vi "测验程序4.vi"() -> ()   [LabVIEW 2017]
uses:
  <vilib>/userdefined/High Color/IMAQdx.ctl
  <vilib>/Platform/TimedLoop/XDataNode/timing_clust.ctl
  <vilib>/Platform/TimedLoop/XDataNode/nitl_modes.ctl
  <vilib>/Platform/TimedLoop/XDataNode/wakeup.ctl
  <vilib>/myRIO/Common/Instrument Driver Framework/myRIO v1.0/UART/vis/myRIO v1.0 Close UART.vi
  <vilib>/FPGAPlugInAG/myRIO-1900/niLvFpga_Open_myRIO-1900.vi
  <vilib>/rvi/interface/common/dynamic/niFpgaDynamicAddResources.vi
  <vilib>/myRIO/Common/Instrument Driver Framework/Utilities/vis/FPGA Ref Manager.vi
  <vilib>/Utility/error.llb/Error Cluster From Error Code.vi
  <vilib>/myRIO/Common/Instrument Driver Framework/Utilities/vis/Ref Counter.vi
  <vilib>/rvi/errors/niLvFpgaAdjustHostInterfaceError.vi
  <vilib>/FPGAPlugInAG/Dynamic/niLvFpga_Close_Dynamic.vi
  <vilib>/myRIO/Common/Instrument Driver Framework/myRIO v1.0/myRIO v1.0 Reset FPGA.vi
  <vilib>/myRIO/Common/Instrument Driver Framework/myRIO v1.0/IRQ/vis/myRIO v1.0 IRQ Info FGV.vi
  <vilib>/myRIO/Common/Instrument Driver Framework/myRIO v1.0/IRQ/vis/myRIO v1.0 Timer IRQ Info FGV.vi
  <vilib>/myRIO/Common/Instrument Driver Framework/myRIO v1.0/IRQ/vis/myRIO v1.0 ISR Agent.vi
  <vilib>/Platform/TimedLoop/XDataNode/XDataNode.xnode
  <vilib>/rvi/interface/nirviOpenFPGA/nirviOpenFPGA.xnode
  <vilib>/rvi/interface/nirviReadWriteControl/nirviReadWriteControl.xnode
  <vilib>/rvi/interface/nirviCloseFPGA/nirviCloseFPGA.xnode
  <vilib>/Platform/TimedLoop/XDataNode/XDNodeRunTimeDep.lvlib
  <vilib>/myRIO/Instrument Drivers/Utilities/Utilities.lvlib
  NiFpgaLv.dll
  <vilib>/rvi/interface/Simulation/niFpgaSimulationCallBeginRW.vi
  <vilib>/vision/driver/NI_Vision_Acquisition_Software.lvlib
  <vilib>/vision/NI_Vision_Development_Module.lvlib
panel:
  in  "Reset":bool
  in  "停止":bool
  out "数量":i32[](array[numeric])
  out "大小":dbl[](array[numeric])
  in  "保留图像？":bool
  in  "停止 2":bool
  out "货物类型":dbl
  in  "初始步态":u16
  in  "开始":bool
  in  "思币得":i32=60
  out "QTI":bool
  out "当前步态":u16
  out "超声波":u32[](array[numeric])
  # "4小蓝"
  # "3小红"
  # "2大蓝"
  # "100000"
  # "1大红"
  # "70000"
  # "0异常"
  # "14600夹取高度"
  # "25000"
  # "700夹住"
  # "-1010"
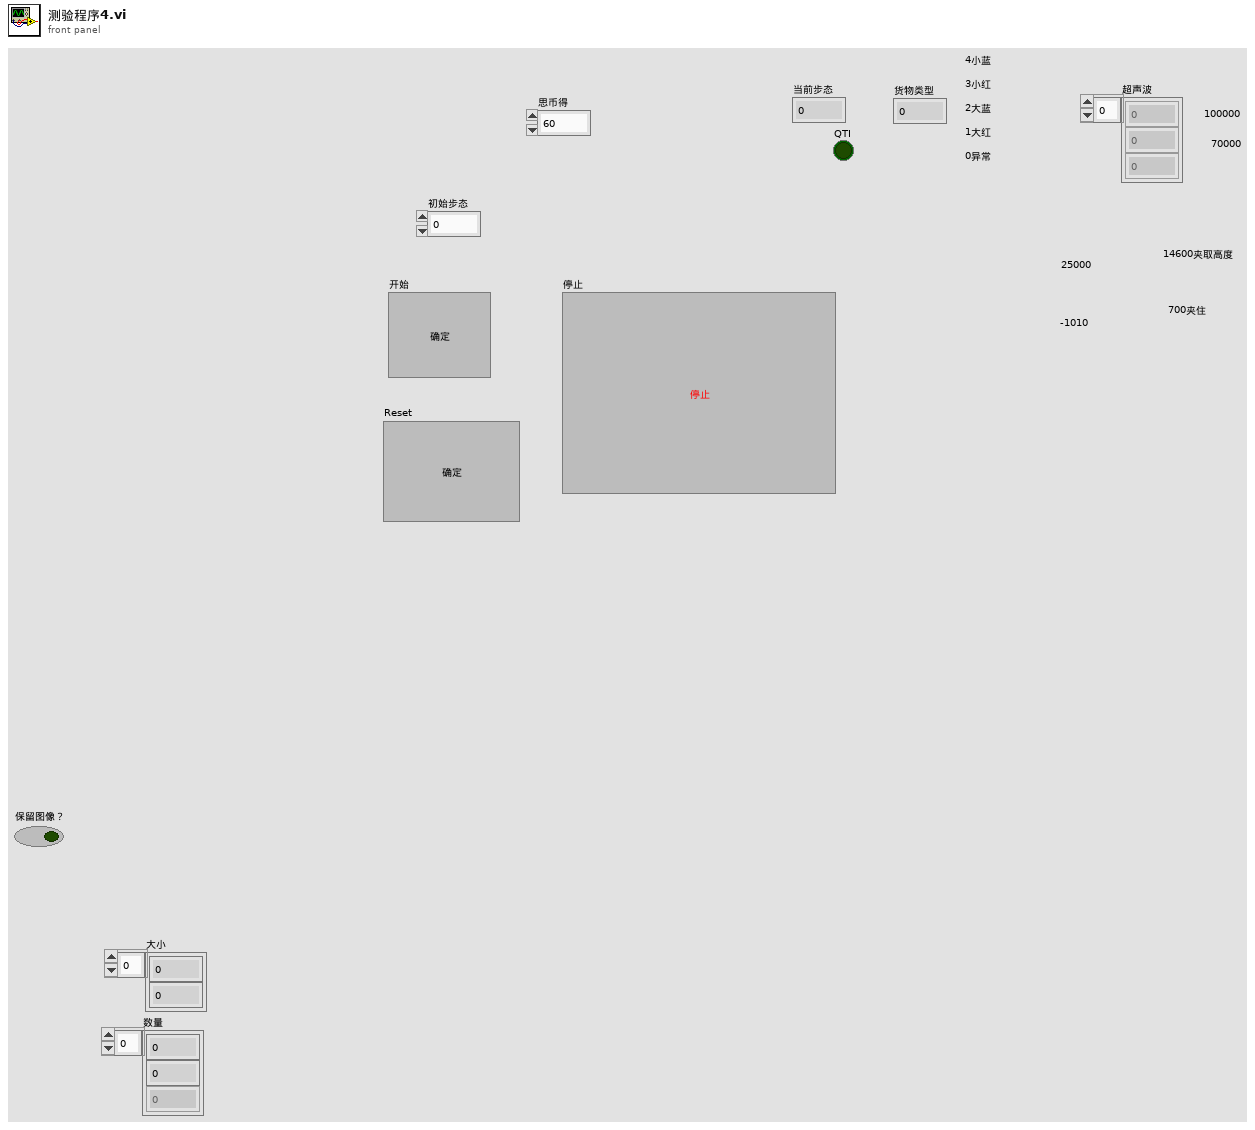
[diagram p1: front panel]
types:
  T1 = typedef "IMAQdx.ctl" = refnum<k21>
  T2 = typedef "IMAQ Image.ctl" = refnum<image>
  T3 = typedef "XDNodeRunTimeDep.lvlib/timing_clust.ctl" = cluster{"Expected End [f-1]":u64, "Actual End [f-1]":u64, "Finished Late? [f-1]":bool, "Expected End [i-1]":u64, "Actual End [i-1]":u64, "Finished Late? [i-1]":bool, "Expected Start [i]":u64, "Actual Start [i]":u64, "Expected Start [f]":u64, "Actual Start [f]":u64, "Source Name":string, "Structure Name":string, "Period":i64, "Deadline":i64, "Offset":i64, "Start":i64, "Priority":i32, "Timeout":i32, "Mode":T4, "Wakeup Reason":T5, "Error":errorcluster, "Source Type":string, "Secondary Source Type":string, "Global End Time":u64, "Global Start Time":u64, "Frame Duration":u64, "Iteration Duration":u64, "Assigned CPU":i32, "I/O Scan Engine Mode":u32}
  T4 = typedef "XDNodeRunTimeDep.lvlib/nitl_modes.ctl" = enum32{"No Change", "Process missed periods, maintain original phase", "Discard missed periods, maintain original phase", "Process missed periods, ignore original phase", "Discard missed periods, ignore original phase"}
  T5 = typedef "XDNodeRunTimeDep.lvlib/wakeup.ctl" = enum32{"Normal", "Aborted", "Asynchronous wakeup", "Timing source error", "Timed loop error", "Timeout"}
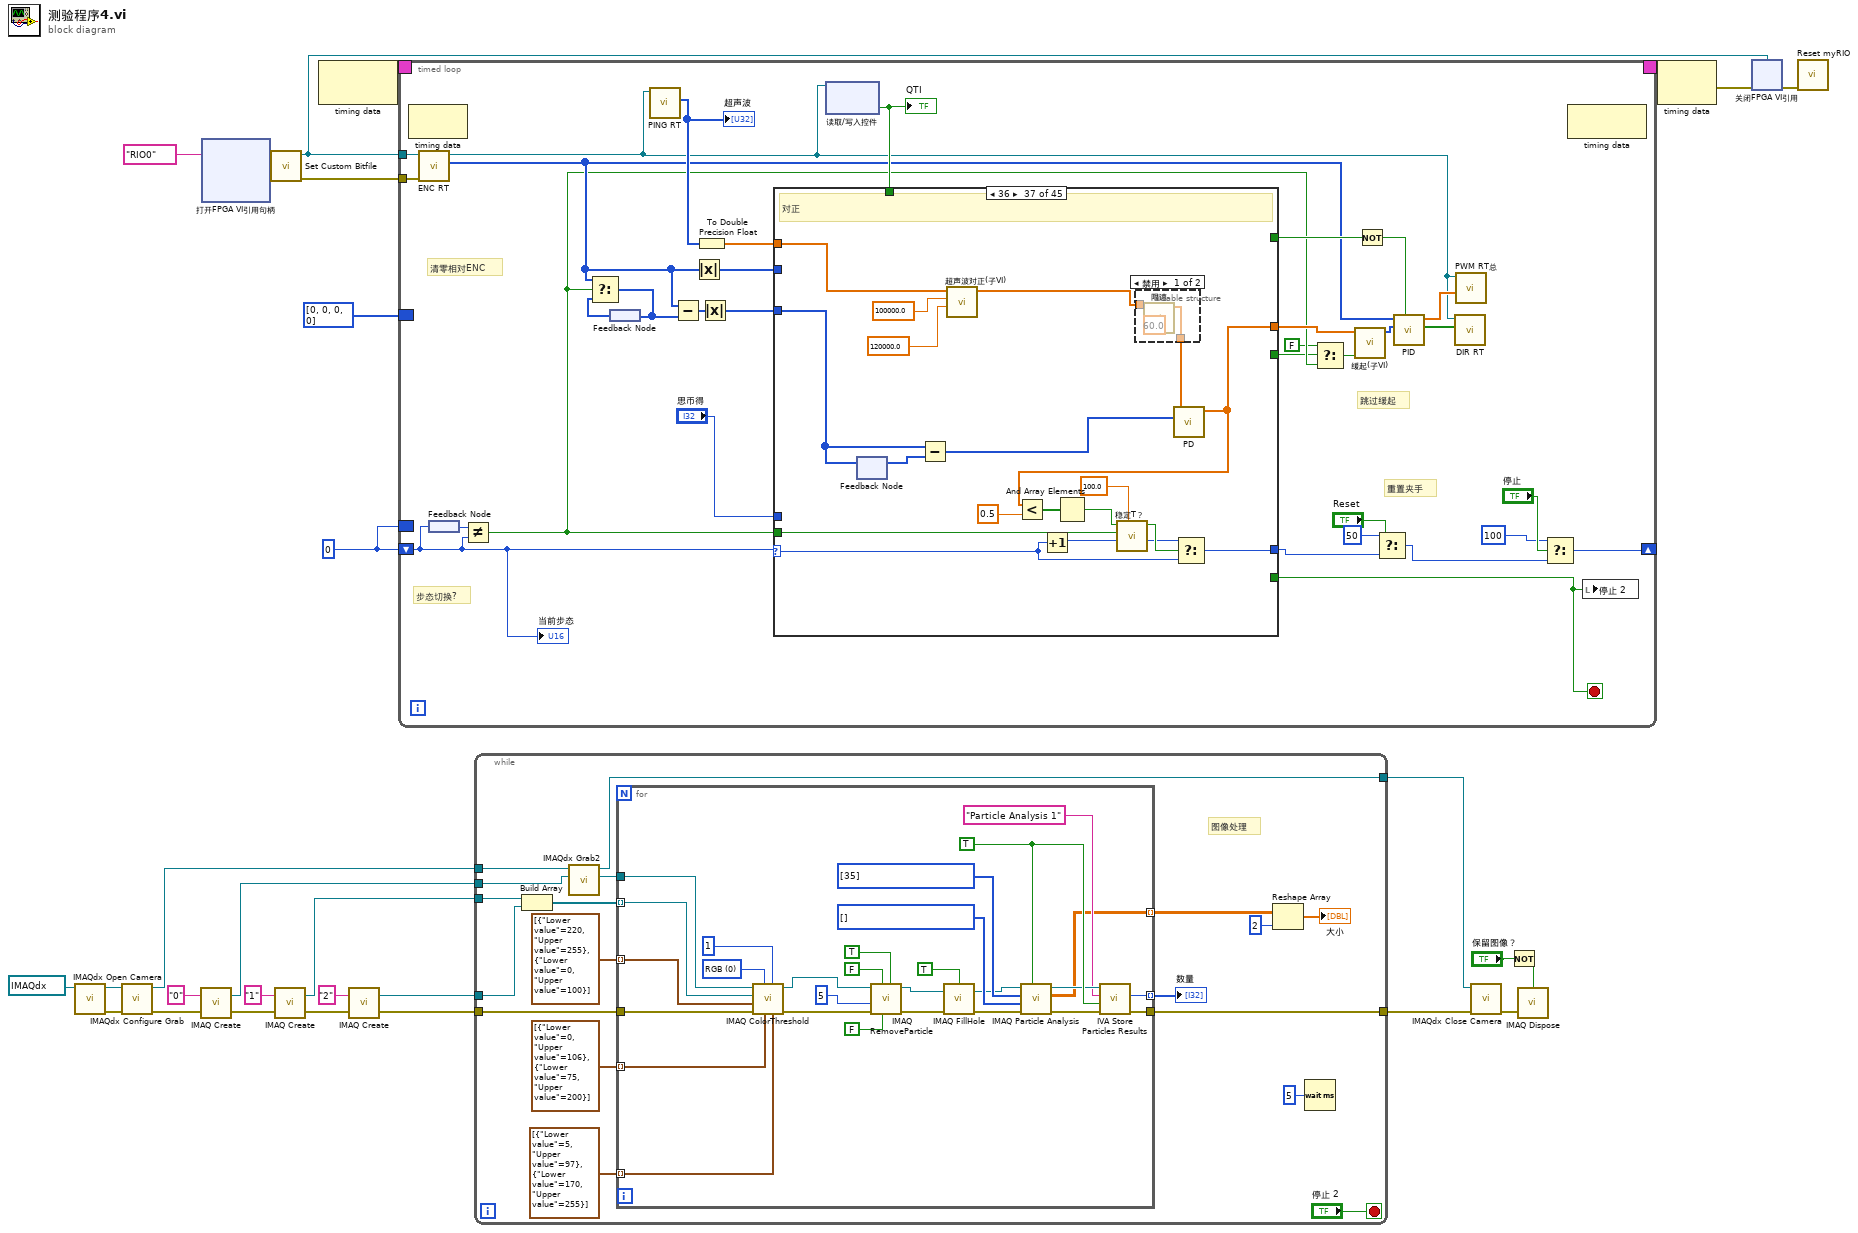
[diagram p0: block diagram]
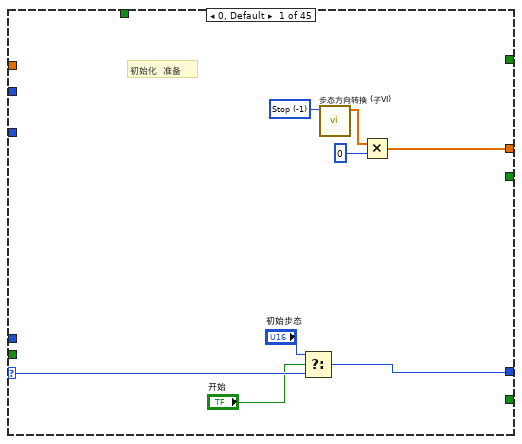
[diagram p2: hidden frame]
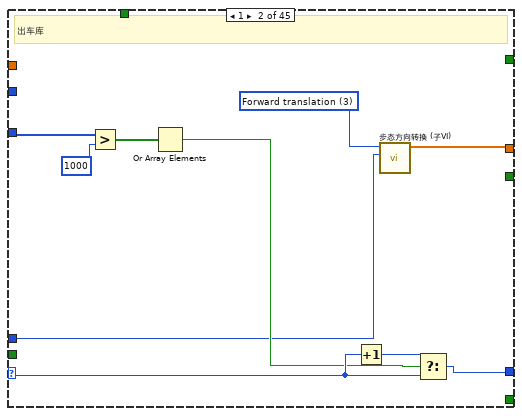
[diagram p3: hidden frame]
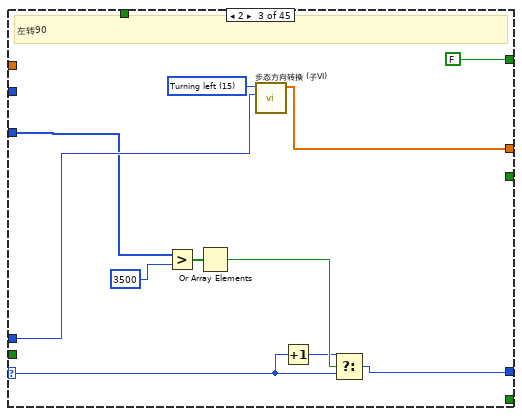
[diagram p4: hidden frame]
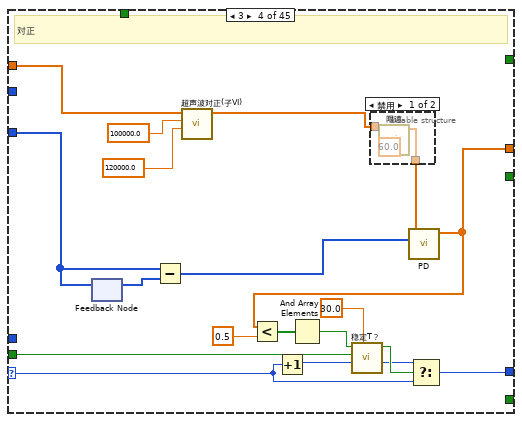
[diagram p5: hidden frame]
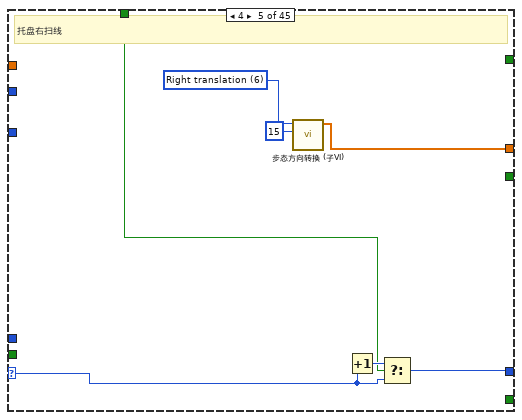
[diagram p7: hidden frame]
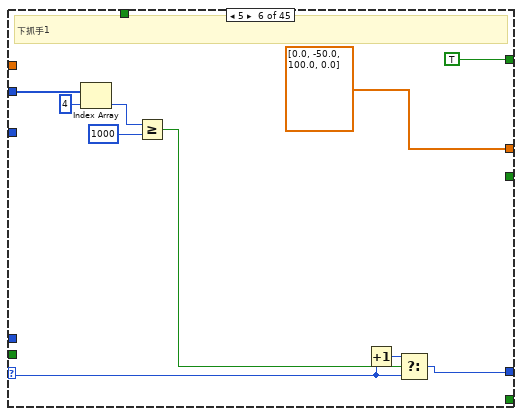
[diagram p8: hidden frame]
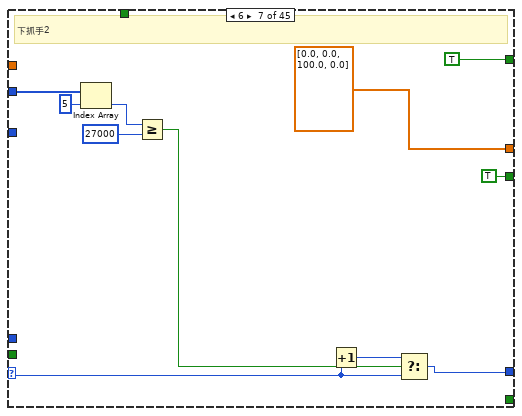
[diagram p9: hidden frame]
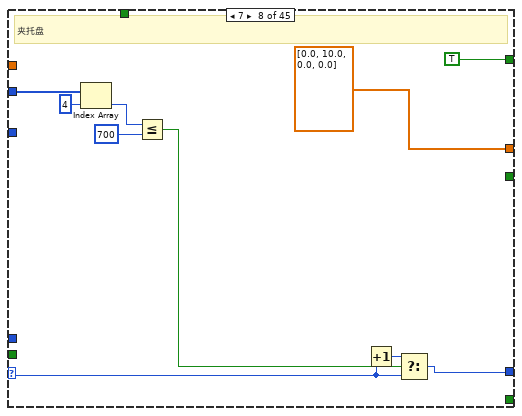
[diagram p10: hidden frame]
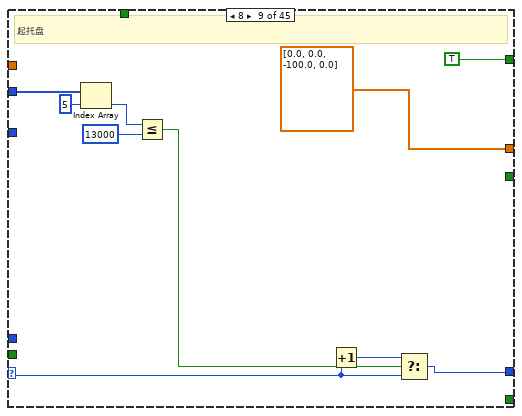
[diagram p11: hidden frame]
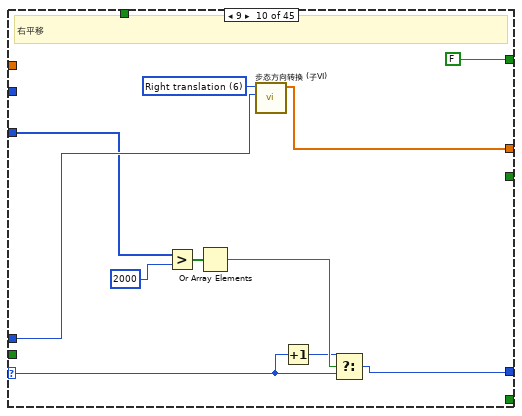
[diagram p12: hidden frame]
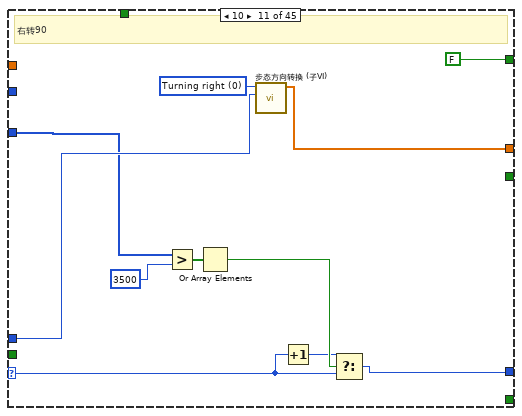
[diagram p13: hidden frame]
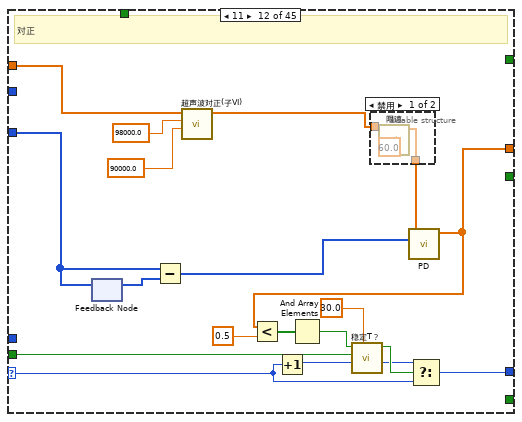
[diagram p14: hidden frame]
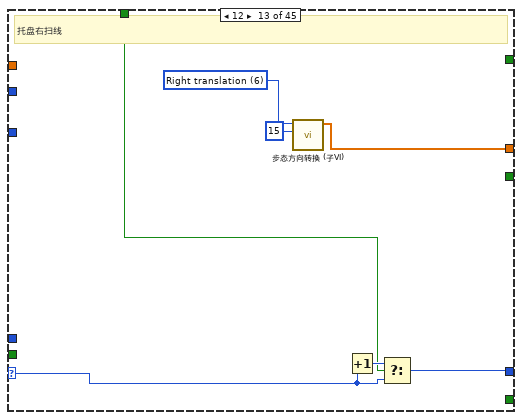
[diagram p16: hidden frame]
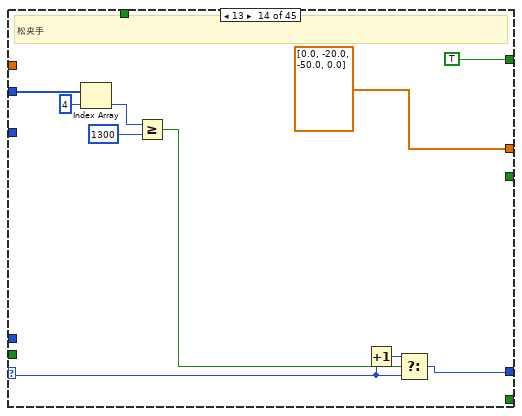
[diagram p17: hidden frame]
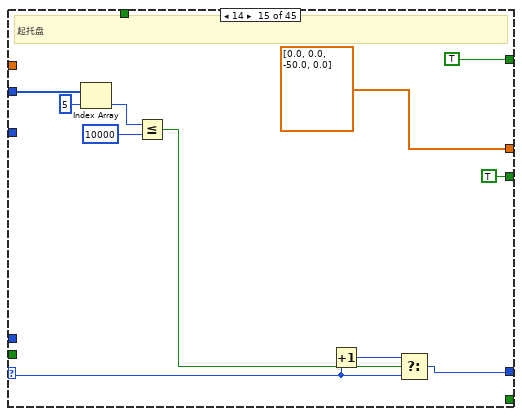
[diagram p18: hidden frame]
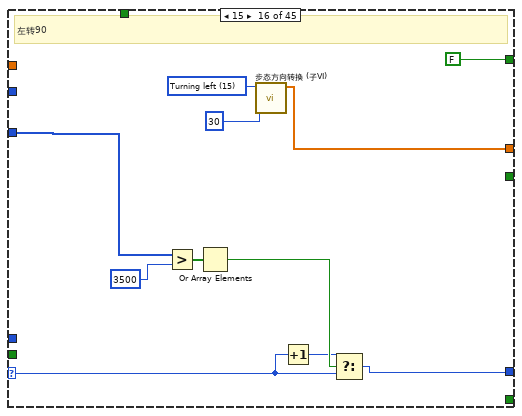
[diagram p19: hidden frame]
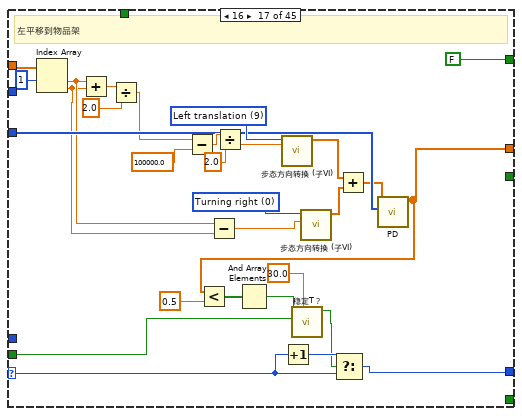
[diagram p20: hidden frame]
diagram:
  w28 = u16 0 ("初始步态")
  n1 = call <vilib>:"IMAQdx Open Camera.vi"("Session In"=T1 "cam0") -> ("error out"=w15:errorcluster, "Session Out"=w14:T1)  [unwired: 9 in]
  n2 = call <vilib>:"IMAQdx Configure Grab.vi"("error in"=w15, "Session In"=w14) -> ("error out"=w12:errorcluster, "Session Out"=w19:T1)  [unwired: 8 in]
  n3 = call "IMAQ Create"("Image Name"="0", "error in (no error)"=w12) -> ("New Image"=w17:T2, "error out"=w10:errorcluster)  [unwired: 3 in]
  n4 = xnode "打开FPGA VI引用句柄"("资源名称"=tag "RIO0") -> ("FPGA VI引用输出"=w24:refnum<k20>, "错误输出"=w23:errorcluster)  [unwired: 1 in]
  n5 = call <vilib>:"Set Custom Bitfile.vi"("error in (no error)"=w23, "Custom FPGA Reference In"=w24) -> ("error out"=w22:errorcluster, "Custom FPGA Reference Out"=w20:refnum<k20>)  [unwired: 8 in]
  n6 = call "IMAQ Create"("Image Name"="1", "error in (no error)"=w10) -> ("New Image"=w7:T2, "error out"=w8:errorcluster)  [unwired: 3 in]
  n7 = node-c288() -> (w30:T3)  [unwired: 1 in]
  n8 = call "IMAQ Create"("Image Name"="2", "error in (no error)"=w8) -> ("New Image"=w6:T2, "error out"=w5:errorcluster)  [unwired: 3 in]
  n9 = timed-loop {
    timing: w30 -> [_]
    timing-out: [_] -> w29
    shift-right: [w42] -> _
    shift-left: w28 -> [w31]
    border: w28 -> [_]
    border: i32[] [0, 0, 0, 0] ("ENC") -> [_]
    tunnel: w22 -> [w60]
    tunnel: w20 -> [w57]
    stop <- w43 stop-if-true
    # "重置夹手"
    # "跳过缓起"
    # "步态切换?"
    # "清零相对ENC"
    n10 = node-c288() -> ()  [unwired: 1 in, 1 out]
    n11 = call "ENC RT.vi"("错误输入（无错误）"=w60, "Custom FPGA Reference Out"=w57) -> ("ENC"=w47:i32[], "FPGA VI引用输出"=w45:refnum<k20>)  [unwired: 7 in, 1 out]
    n12 = feedback-in #1(w31) -> ()
    n13 = feedback #1() -> (w61:u16)
    n14 = Not Equal?(x=w61, y=w31) -> (x != y?=w35:bool)
    n15 = feedback #2() -> (w59:i32[])
    n16 = Select(t=w47, s=w35, f=w59) -> (s? t:f=w44:i32[])
    n17 = feedback-in #2(w44) -> ()
    n18 = call "PING RT.vi"("引用句柄输入"=w45) -> ("PING"=w51:u32[])  [unwired: 8 in, 2 out]
    "超声波" <- w51
    n19 = Subtract(x=w47, y=w44) -> (x-y=w52:i32[])
    n20 = Absolute Value(x=w47) -> (abs(x)=w46:i32[])
    n21 = To Double Precision Float(number=w51) -> (double precision float=w50:dbl[])
    n22 = Absolute Value(x=w52) -> (abs(x)=w48:i32[])
    n23 = xnode "读取/写入控件"("FPGA VI引用输入"=w45) -> ("QTI"=w49:bool)  [unwired: 1 in, 2 out]
    "QTI" <- w49
    n24 = case shown="36" w31 {
      selector: w31 -> [w68 w74 w85 w108 w118 w128 w140 w150 w160 w166 w177 w200 w210 w221 w232 w239 w272 w278 w286 w310 w316 w327 w337 w347 w353 w387 w393 w401 w423 w429 w440 w451 w462 w472 w479 w488 w511 w526 w536 w545 w557 w568 w579 w587 w599]
      tunnel: [w69 w81 w86 w102 w119 dbl[] [0.0, -50.0, 100.0, 0.0] ("输出") dbl[] [0.0, 0.0, 100.0, 0.0] ("输出") dbl[] [0.0, 10.0, 0.0, 0.0] ("输出") dbl[] [0.0, 0.0, -100.0, 0.0] ("输出") w167 w178 w194 w211 dbl[] [0.0, -20.0, -50.0, 0.0] ("输出") dbl[] [0.0, 0.0, -50.0, 0.0] ("输出") w240 w260 w279 w287 w297 w317 dbl[] [0.0, 0.0, 50.0, 0.0] ("输出") dbl[] [0.0, 10.0, 0.0, 0.0] ("输出") dbl[] [0.0, 0.0, -50.0, 0.0] ("输出") w354 w375 w394 w402 w411 w430 dbl[] [0.0, -10.0, 0.0, 0.0] ("输出") dbl[] [0.0, 0.0, 100.0, 0.0] ("输出") dbl[] [0.0, 10.0, 0.0, 0.0] ("输出") dbl[] [0.0, 0.0, -100.0, 0.0] ("输出") w480 w495 w505 dbl[] [0.0, 0.0, 100.0, 0.0] ("输出") dbl[] [0.0, -10.0, 0.0, 0.0] ("输出") dbl[] [0.0, 50.0, -100.0, 0.0] ("输出") dbl[] [0.0, 0.0, -100.0, 0.0] ("输出") w566 dbl[] [0.0, 10.0, 0.0, 0.0] ("输出") dbl[] [0.0, 0.0, 0.0, 0.0] ("输出") dbl[] [0.0, 0.0, 0.0, 0.0] ("输出")] -> w56
      tunnel: "思币得" -> [_ w72 w87 _ _ _ _ _ _ w168 w179 _ _ _ _ _ _ _ _ _ _ _ _ _ w355 _ _ _ _ _ _ _ _ _ _ _ _ _ _ _ _ w560 _ _ _]
      tunnel: [w66 w77 w92 w107 w116 w130 w141 w151 w161 w173 w184 w199 w208 w222 w233 w245 w274 w276 w292 w312 w314 w328 w338 w348 w360 w389 w391 w407 w425 w427 w441 w452 w463 w473 w485 w491 w510 w527 w537 w547 w558 w569 w581 w589 w599] -> w39
      tunnel: [_ _ FALSE ("继电器") _ _ TRUE ("继电器") TRUE ("继电器") TRUE ("继电器") TRUE ("继电器") FALSE ("继电器") FALSE ("继电器") _ _ TRUE ("继电器") TRUE ("继电器") FALSE ("继电器") FALSE ("继电器") _ FALSE ("继电器") FALSE ("继电器") _ TRUE ("继电器") TRUE ("继电器") TRUE ("继电器") FALSE ("继电器") FALSE ("继电器") _ FALSE ("继电器") FALSE ("继电器") _ TRUE ("继电器") TRUE ("继电器") TRUE ("继电器") TRUE ("继电器") FALSE ("继电器") _ _ TRUE ("继电器") TRUE ("继电器") TRUE ("继电器") TRUE ("继电器") _ TRUE ("继电器") _ _] -> w54
      tunnel: w48 -> [_ w79 w83 w105 _ _ _ _ _ w164 w175 w197 _ _ _ w237 w266 _ w284 w303 _ _ _ _ w351 w381 _ w399 w417 _ _ _ _ _ w477 w493 w508 _ _ _ _ w562 _ _ _]
      tunnel: w50 -> [_ _ _ w110 _ _ _ _ _ _ _ w202 _ _ _ _ w270 _ _ w308 _ _ _ _ _ w385 _ _ w421 _ _ _ _ _ _ _ w513 _ _ _ _ _ _ _ _]
      tunnel: w35 -> [_ _ _ w97 _ _ _ _ _ _ _ w189 _ _ _ _ w259 _ _ w296 _ _ _ _ _ w374 _ _ w410 _ _ _ _ _ _ _ w500 _ _ _ _ _ _ _ _]
      tunnel: w49 -> [_ _ _ _ w115 _ _ _ _ _ _ _ w207 _ _ _ _ w275 _ _ w313 _ _ _ _ _ w390 _ _ w426 _ _ _ _ _ _ _ _ _ _ _ _ _ _ _]
      tunnel: w46 -> [_ _ _ _ _ w122 w134 w144 w154 _ _ _ _ w215 w226 _ _ _ _ _ _ w321 w331 w341 _ _ _ _ _ _ w434 w445 w456 w466 _ _ _ w520 w530 w539 w551 _ w573 _ _]
      tunnel: [_ _ _ _ _ _ _ _ _ _ _ _ _ _ _ _ _ _ _ _ _ _ _ _ _ _ _ _ _ _ _ _ _ _ _ _ _ _ _ _ _ _ _ _ TRUE ("停止 2")] -> w43
      tunnel: [_ _ _ _ _ _ TRUE ("t") _ _ _ _ _ _ _ TRUE ("t") _ _ _ _ _ _ _ _ _ _ _ _ _ _ _ _ TRUE ("t") TRUE ("t") _ _ _ _ TRUE ("t") _ _ TRUE ("t") _ _ _ _] -> w32
      frame 0, Default {
        w71 = i8 -1 items=["Stop"=-1, "Right translation"=6, "Back translation"=12, "Turning right"=0, "Turning left"=15, "Forward translation"=3, "Left translation"=9, "Gyro rotating"=16] ("Gait")
        # "初始化  准备"
        n25 = Select(t="初始步态", s="开始", f=w68) -> (s? t:f=w66:u16)
        n26 = call "步态方向转换 (子VI).vi"("Gait"=w71) -> ("输出"=w70:dbl[])  [unwired: 10 in]
        n27 = Multiply(x=w70, y=0 ("长度")) -> (x*y=w69:dbl[])
      }
      frame 1 {
        w80 = i8 3 items=["Stop"=-1, "Right translation"=6, "Back translation"=12, "Turning right"=0, "Turning left"=15, "Forward translation"=3, "Left translation"=9, "Gyro rotating"=16] ("Gait")
        # "出车库"
        n28 = Greater?(x=w79, y=1000) -> (0:w76:bool[])
        n29 = Or Array Elements(Boolean array=w76) -> (logical OR=w73:bool)
        n30 = Increment(x=w74) -> (x+1=w75:u16)
        n31 = call "步态方向转换 (子VI).vi"("速度"=w72, "Gait"=w80) -> ("输出"=w81:dbl[])  [unwired: 9 in]
        n32 = Select(t=w75, s=w73, f=w74) -> (s? t:f=w77:u16)
      }
      frame 2 {
        w88 = i8 15 items=["Stop"=-1, "Right translation"=6, "Back translation"=12, "Turning right"=0, "Turning left"=15, "Forward translation"=3, "Left translation"=9, "Gyro rotating"=16] ("Gait")
        # "左转90"
        n33 = Greater?(x=w83, y=3500 ("次数")) -> (0:w90:bool[])
        n34 = Or Array Elements(Boolean array=w90) -> (logical OR=w89:bool)
        n35 = call "步态方向转换 (子VI).vi"("速度"=w87, "Gait"=w88) -> ("输出"=w86:dbl[])  [unwired: 9 in]
        n36 = Increment(x=w85) -> (x+1=w84:u16)
        n37 = Select(t=w84, s=w89, f=w85) -> (s? t:f=w92:u16)
      }
      frame 3 {
        # "对正"
        n38 = feedback-in #3(w105) -> ()
        n39 = feedback #3() -> (w104:i32[])  [unwired: 1 in]
        n40 = Subtract(x=w105, y=w104) -> (x-y=w103:i32[])
        n41 = call "超声波对正(子VI).vi"("LFT"=120000.0, "FWD"=100000.0, "数组输入"=w110) -> ("数组输出"=w109:dbl[])  [unwired: 8 in]
        n42 = Increment(x=w108) -> (x+1=w93:u16)
        n43 = disable-structure shown="禁用" {
          disable-tunnel: w109 -> [w113 w114]
          disable-tunnel: [w111 w114] -> w106
          frame Disabled {
            n44 = call "限速.vi"("最大值"=60.0, "输入"=w113) -> ("数组"=w111:dbl[])  [unwired: 9 in]
          }
          frame Enabled {
          }
        }
        n45 = call "PD.vi"("ENC"=w103, "SET"=w106) -> ("output"=w102:dbl[])  [unwired: 9 in]
        n46 = Less?(x=w102, y=0.5) -> (x < y?=w100:bool[])
        n47 = And Array Elements(Boolean array=w100) -> (logical AND=w99:bool)
        n48 = call "稳定T？.vi"("次数(100)"=30.0, "Reset"=w97, "输入"=w99) -> ("TT？"=w98:bool)  [unwired: 8 in]
        n49 = Select(t=w93, s=w98, f=w108) -> (s? t:f=w107:u16)
      }
      frame 4 {
        w121 = i8 6 items=["Stop"=-1, "Right translation"=6, "Back translation"=12, "Turning right"=0, "Turning left"=15, "Forward translation"=3, "Left translation"=9, "Gyro rotating"=16] ("Gait")
        # "托盘右扫线"
        n50 = call "步态方向转换 (子VI).vi"("速度"=15, "Gait"=w121) -> ("输出"=w119:dbl[])  [unwired: 9 in]
        n51 = Increment(x=w118) -> (x+1=w117:u16)
        n52 = Select(t=w117, s=w115, f=w118) -> (s? t:f=w116:u16)
      }
      frame 5 {
        # "下抓手1"
        n53 = Index Array(array=w122, index=4 ("索引")) -> (element=w125:i32)
        n54 = Greater Or Equal?(x=w125, y=1000) -> (x >= y?=w123:bool)
        n55 = Increment(x=w128) -> (x+1=w129:u16)
        n56 = Select(t=w129, s=w123, f=w128) -> (s? t:f=w130:u16)
      }
      frame 6 {
        # "下抓手2"
        n57 = Index Array(array=w134, index=5 ("索引")) -> (element=w137:i32)
        n58 = Greater Or Equal?(x=w137, y=27000) -> (x >= y?=w135:bool)
        n59 = Increment(x=w140) -> (x+1=w133:u16)
        n60 = Select(t=w133, s=w135, f=w140) -> (s? t:f=w141:u16)
      }
      frame 7 {
        # "夹托盘"
        n61 = Index Array(array=w144, index=4 ("索引")) -> (element=w147:i32)
        n62 = Less Or Equal?(x=w147, y=700) -> (x <= y?=w145:bool)
        n63 = Increment(x=w150) -> (x+1=w143:u16)
        n64 = Select(t=w143, s=w145, f=w150) -> (s? t:f=w151:u16)
      }
      frame 8 {
        # "起托盘"
        n65 = Index Array(array=w154, index=5 ("索引")) -> (element=w157:i32)
        n66 = Less Or Equal?(x=w157, y=13000) -> (x <= y?=w155:bool)
        n67 = Increment(x=w160) -> (x+1=w153:u16)
        n68 = Select(t=w153, s=w155, f=w160) -> (s? t:f=w161:u16)
      }
      frame 9 {
        w169 = i8 6 items=["Stop"=-1, "Right translation"=6, "Back translation"=12, "Turning right"=0, "Turning left"=15, "Forward translation"=3, "Left translation"=9, "Gyro rotating"=16] ("Gait")
        # "右平移"
        n69 = Greater?(x=w164, y=2000 ("次数")) -> (0:w171:bool[])
        n70 = Or Array Elements(Boolean array=w171) -> (logical OR=w170:bool)
        n71 = call "步态方向转换 (子VI).vi"("速度"=w168, "Gait"=w169) -> ("输出"=w167:dbl[])  [unwired: 9 in]
        n72 = Increment(x=w166) -> (x+1=w165:u16)
        n73 = Select(t=w165, s=w170, f=w166) -> (s? t:f=w173:u16)
      }
      frame 10 {
        w180 = i8 0 items=["Stop"=-1, "Right translation"=6, "Back translation"=12, "Turning right"=0, "Turning left"=15, "Forward translation"=3, "Left translation"=9, "Gyro rotating"=16] ("Gait")
        # "右转90"
        n74 = Greater?(x=w175, y=3500 ("次数")) -> (0:w182:bool[])
        n75 = Or Array Elements(Boolean array=w182) -> (logical OR=w181:bool)
        n76 = call "步态方向转换 (子VI).vi"("速度"=w179, "Gait"=w180) -> ("输出"=w178:dbl[])  [unwired: 9 in]
        n77 = Increment(x=w177) -> (x+1=w176:u16)
        n78 = Select(t=w176, s=w181, f=w177) -> (s? t:f=w184:u16)
      }
      frame 11 {
        # "对正"
        n79 = feedback-in #4(w197) -> ()
        n80 = feedback #4() -> (w196:i32[])  [unwired: 1 in]
        n81 = Subtract(x=w197, y=w196) -> (x-y=w195:i32[])
        n82 = call "超声波对正(子VI).vi"("LFT"=90000.0, "FWD"=98000.0, "数组输入"=w202) -> ("数组输出"=w201:dbl[])  [unwired: 8 in]
        n83 = Increment(x=w200) -> (x+1=w185:u16)
        n84 = disable-structure shown="禁用" {
          disable-tunnel: w201 -> [w205 w206]
          disable-tunnel: [w203 w206] -> w198
          frame Disabled {
            n85 = call "限速.vi"("最大值"=60.0, "输入"=w205) -> ("数组"=w203:dbl[])  [unwired: 9 in]
          }
          frame Enabled {
          }
        }
        n86 = call "PD.vi"("ENC"=w195, "SET"=w198) -> ("output"=w194:dbl[])  [unwired: 9 in]
        n87 = Less?(x=w194, y=0.5) -> (x < y?=w192:bool[])
        n88 = And Array Elements(Boolean array=w192) -> (logical AND=w191:bool)
        n89 = call "稳定T？.vi"("次数(100)"=30.0, "Reset"=w189, "输入"=w191) -> ("TT？"=w190:bool)  [unwired: 8 in]
        n90 = Select(t=w185, s=w190, f=w200) -> (s? t:f=w199:u16)
      }
      frame 12 {
        w213 = i8 6 items=["Stop"=-1, "Right translation"=6, "Back translation"=12, "Turning right"=0, "Turning left"=15, "Forward translation"=3, "Left translation"=9, "Gyro rotating"=16] ("Gait")
        # "托盘右扫线"
        n91 = call "步态方向转换 (子VI).vi"("速度"=15, "Gait"=w213) -> ("输出"=w211:dbl[])  [unwired: 9 in]
        n92 = Increment(x=w210) -> (x+1=w209:u16)
        n93 = Select(t=w209, s=w207, f=w210) -> (s? t:f=w208:u16)
      }
      frame 13 {
        # "松夹手"
        n94 = Index Array(array=w215, index=4 ("索引")) -> (element=w218:i32)
        n95 = Greater Or Equal?(x=w218, y=1300) -> (x >= y?=w216:bool)
        n96 = Increment(x=w221) -> (x+1=w214:u16)
        n97 = Select(t=w214, s=w216, f=w221) -> (s? t:f=w222:u16)
      }
      frame 14 {
        # "起托盘"
        n98 = Index Array(array=w226, index=5 ("索引")) -> (element=w229:i32)
        n99 = Less Or Equal?(x=w229, y=10000) -> (x <= y?=w227:bool)
        n100 = Increment(x=w232) -> (x+1=w225:u16)
        n101 = Select(t=w225, s=w227, f=w232) -> (s? t:f=w233:u16)
      }
      frame 15 {
        w241 = i8 15 items=["Stop"=-1, "Right translation"=6, "Back translation"=12, "Turning right"=0, "Turning left"=15, "Forward translation"=3, "Left translation"=9, "Gyro rotating"=16] ("Gait")
        # "左转90"
        n102 = Greater?(x=w237, y=3500 ("次数")) -> (0:w243:bool[])
        n103 = Or Array Elements(Boolean array=w243) -> (logical OR=w242:bool)
        n104 = call "步态方向转换 (子VI).vi"("速度"=30, "Gait"=w241) -> ("输出"=w240:dbl[])  [unwired: 9 in]
        n105 = Increment(x=w239) -> (x+1=w238:u16)
        n106 = Select(t=w238, s=w242, f=w239) -> (s? t:f=w245:u16)
      }
      frame 16 {
        w251 = i8 0 items=["Stop"=-1, "Right translation"=6, "Back translation"=12, "Turning right"=0, "Turning left"=15, "Forward translation"=3, "Left translation"=9, "Gyro rotating"=16] ("Gait")
        w269 = i8 9 items=["Stop"=-1, "Right translation"=6, "Back translation"=12, "Turning right"=0, "Turning left"=15, "Forward translation"=3, "Left translation"=9, "Gyro rotating"=16] ("Gait")
        # "左平移到物品架"
        n107 = Index Array(array=w270, index #1=1 ("索引")) -> (element #1=w250:dbl, element #2=w249:dbl)  [unwired: 1 in]
        n108 = Add(x=w250, y=w249) -> (x+y=w255:dbl)
        n109 = Divide(x=w255, y=2.0) -> (x/y=w253:dbl)
        n110 = Subtract(x=w253, y=100000.0) -> (x-y=w268:dbl)
        n111 = Subtract(x=w250, y=w249) -> (x-y=w252:dbl)
        n112 = Divide(x=w268, y=2.0 ("x")) -> (x/y=w258:dbl)
        n113 = call "步态方向转换 (子VI).vi"("速度"=w258, "Gait"=w269) -> ("输出"=w248:dbl[])  [unwired: 9 in]
        n114 = Increment(x=w272) -> (x+1=w271:u16)
        n115 = call "步态方向转换 (子VI).vi"("速度"=w252, "Gait"=w251) -> ("输出"=w247:dbl[])  [unwired: 9 in]
        n116 = Add(x=w248, y=w247) -> (x+y=w246:dbl[])
        n117 = call "PD.vi"("ENC"=w266, "SET"=w246) -> ("output"=w260:dbl[])  [unwired: 9 in]
        n118 = Less?(x=w260, y=0.5) -> (x < y?=w264:bool[])
        n119 = And Array Elements(Boolean array=w264) -> (logical AND=w263:bool)
        n120 = call "稳定T？.vi"("次数(100)"=30.0, "Reset"=w259, "输入"=w263) -> ("TT？"=w261:bool)  [unwired: 8 in]
        n121 = Select(t=w271, s=w261, f=w272) -> (s? t:f=w274:u16)
      }
      frame 17 {
        w281 = i8 12 items=["Stop"=-1, "Right translation"=6, "Back translation"=12, "Turning right"=0, "Turning left"=15, "Forward translation"=3, "Left translation"=9, "Gyro rotating"=16] ("Gait")
        # "货物架后扫线"
        n122 = call "步态方向转换 (子VI).vi"("速度"=15, "Gait"=w281) -> ("输出"=w279:dbl[])  [unwired: 9 in]
        n123 = Increment(x=w278) -> (x+1=w277:u16)
        n124 = Select(t=w277, s=w275, f=w278) -> (s? t:f=w276:u16)
      }
      frame 18 {
        w288 = i8 15 items=["Stop"=-1, "Right translation"=6, "Back translation"=12, "Turning right"=0, "Turning left"=15, "Forward translation"=3, "Left translation"=9, "Gyro rotating"=16] ("Gait")
        # "左转90"
        n125 = Greater?(x=w284, y=3500 ("次数")) -> (0:w290:bool[])
        n126 = Or Array Elements(Boolean array=w290) -> (logical OR=w289:bool)
        n127 = call "步态方向转换 (子VI).vi"("速度"=30, "Gait"=w288) -> ("输出"=w287:dbl[])  [unwired: 9 in]
        n128 = Increment(x=w286) -> (x+1=w285:u16)
        n129 = Select(t=w285, s=w289, f=w286) -> (s? t:f=w292:u16)
      }
      frame 19 {
        w307 = i8 3 items=["Stop"=-1, "Right translation"=6, "Back translation"=12, "Turning right"=0, "Turning left"=15, "Forward translation"=3, "Left translation"=9, "Gyro rotating"=16] ("Gait")
        # "物品架前对正"
        n130 = Index Array(array=w308) -> (element=w293:dbl)  [unwired: 1 in]
        n131 = Subtract(x=w293, y=95000.0) -> (x-y=w306:dbl)
        n132 = Divide(x=w306, y=2.0 ("x")) -> (x/y=w295:dbl)
        n133 = Increment(x=w310) -> (x+1=w309:u16)
        n134 = call "步态方向转换 (子VI).vi"("速度"=w295, "Gait"=w307) -> ("输出"=w305:dbl[])  [unwired: 9 in]
        n135 = call "PD.vi"("ENC"=w303, "SET"=w305) -> ("output"=w297:dbl[])  [unwired: 9 in]
        n136 = Less?(x=w297, y=0.5) -> (x < y?=w301:bool[])
        n137 = And Array Elements(Boolean array=w301) -> (logical AND=w300:bool)
        n138 = call "稳定T？.vi"("次数(100)"=30.0, "Reset"=w296, "输入"=w300) -> ("TT？"=w298:bool)  [unwired: 8 in]
        n139 = Select(t=w309, s=w298, f=w310) -> (s? t:f=w312:u16)
      }
      frame 20 {
        w319 = i8 6 items=["Stop"=-1, "Right translation"=6, "Back translation"=12, "Turning right"=0, "Turning left"=15, "Forward translation"=3, "Left translation"=9, "Gyro rotating"=16] ("Gait")
        # "货物架右扫线"
        n140 = call "步态方向转换 (子VI).vi"("速度"=15, "Gait"=w319) -> ("输出"=w317:dbl[])  [unwired: 9 in]
        n141 = Increment(x=w316) -> (x+1=w315:u16)
        n142 = Select(t=w315, s=w313, f=w316) -> (s? t:f=w314:u16)
      }
      frame 21 {
        # "下抓手"
        n143 = Index Array(array=w321, index=5 ("索引")) -> (element=w324:i32)
        n144 = Greater Or Equal?(x=w324, y=14600) -> (x >= y?=w322:bool)
        n145 = Increment(x=w327) -> (x+1=w320:u16)
        n146 = Select(t=w320, s=w322, f=w327) -> (s? t:f=w328:u16)
      }
      frame 22 {
        # "抓取"
        n147 = Index Array(array=w331, index=4 ("索引")) -> (element=w334:i32)
        n148 = Less Or Equal?(x=w334, y=180) -> (x <= y?=w332:bool)
        n149 = Increment(x=w337) -> (x+1=w330:u16)
        n150 = Select(t=w330, s=w332, f=w337) -> (s? t:f=w338:u16)
      }
      frame 23 {
        # "抬升"
        n151 = Index Array(array=w341, index=5 ("索引")) -> (element=w344:i32)
        n152 = Less Or Equal?(x=w344, y=11800) -> (x <= y?=w342:bool)
        n153 = Increment(x=w347) -> (x+1=w340:u16)
        n154 = Select(t=w340, s=w342, f=w347) -> (s? t:f=w348:u16)
      }
      frame 24 {
        w356 = i8 15 items=["Stop"=-1, "Right translation"=6, "Back translation"=12, "Turning right"=0, "Turning left"=15, "Forward translation"=3, "Left translation"=9, "Gyro rotating"=16] ("Gait")
        # "左转90"
        n155 = Greater?(x=w351, y=3500 ("次数")) -> (0:w358:bool[])
        n156 = Or Array Elements(Boolean array=w358) -> (logical OR=w357:bool)
        n157 = call "步态方向转换 (子VI).vi"("速度"=w355, "Gait"=w356) -> ("输出"=w354:dbl[])  [unwired: 9 in]
        n158 = Increment(x=w353) -> (x+1=w352:u16)
        n159 = Select(t=w352, s=w357, f=w353) -> (s? t:f=w360:u16)
      }
      frame 25 {
        w366 = i8 0 items=["Stop"=-1, "Right translation"=6, "Back translation"=12, "Turning right"=0, "Turning left"=15, "Forward translation"=3, "Left translation"=9, "Gyro rotating"=16] ("Gait")
        w384 = i8 9 items=["Stop"=-1, "Right translation"=6, "Back translation"=12, "Turning right"=0, "Turning left"=15, "Forward translation"=3, "Left translation"=9, "Gyro rotating"=16] ("Gait")
        # "左平移到组装架"
        n160 = Index Array(array=w385, index #1=1 ("索引")) -> (element #1=w365:dbl, element #2=w364:dbl)  [unwired: 1 in]
        n161 = Add(x=w365, y=w364) -> (x+y=w370:dbl)
        n162 = Divide(x=w370, y=2.0) -> (x/y=w368:dbl)
        n163 = Subtract(x=w368, y=95000.0) -> (x-y=w383:dbl)
        n164 = Subtract(x=w365, y=w364) -> (x-y=w367:dbl)
        n165 = Divide(x=w383, y=2.0 ("x")) -> (x/y=w373:dbl)
        n166 = call "步态方向转换 (子VI).vi"("速度"=w373, "Gait"=w384) -> ("输出"=w363:dbl[])  [unwired: 9 in]
        n167 = Increment(x=w387) -> (x+1=w386:u16)
        n168 = call "步态方向转换 (子VI).vi"("速度"=w367, "Gait"=w366) -> ("输出"=w362:dbl[])  [unwired: 9 in]
        n169 = Add(x=w363, y=w362) -> (x+y=w361:dbl[])
        n170 = call "PD.vi"("ENC"=w381, "SET"=w361) -> ("output"=w375:dbl[])  [unwired: 9 in]
        n171 = Less?(x=w375, y=0.5) -> (x < y?=w379:bool[])
        n172 = And Array Elements(Boolean array=w379) -> (logical AND=w378:bool)
        n173 = call "稳定T？.vi"("次数(100)"=30.0, "Reset"=w374, "输入"=w378) -> ("TT？"=w376:bool)  [unwired: 8 in]
        n174 = Select(t=w386, s=w376, f=w387) -> (s? t:f=w389:u16)
      }
      frame 26 {
        w396 = i8 12 items=["Stop"=-1, "Right translation"=6, "Back translation"=12, "Turning right"=0, "Turning left"=15, "Forward translation"=3, "Left translation"=9, "Gyro rotating"=16] ("Gait")
        # "组装台后扫线"
        n175 = call "步态方向转换 (子VI).vi"("速度"=15, "Gait"=w396) -> ("输出"=w394:dbl[])  [unwired: 9 in]
        n176 = Increment(x=w393) -> (x+1=w392:u16)
        n177 = Select(t=w392, s=w390, f=w393) -> (s? t:f=w391:u16)
      }
      frame 27 {
        w403 = i8 15 items=["Stop"=-1, "Right translation"=6, "Back translation"=12, "Turning right"=0, "Turning left"=15, "Forward translation"=3, "Left translation"=9, "Gyro rotating"=16] ("Gait")
        # "左转90"
        n178 = Greater?(x=w399, y=3500 ("次数")) -> (0:w405:bool[])
        n179 = Or Array Elements(Boolean array=w405) -> (logical OR=w404:bool)
        n180 = call "步态方向转换 (子VI).vi"("速度"=30, "Gait"=w403) -> ("输出"=w402:dbl[])  [unwired: 9 in]
        n181 = Increment(x=w401) -> (x+1=w400:u16)
        n182 = Select(t=w400, s=w404, f=w401) -> (s? t:f=w407:u16)
      }
      frame 28 {
        w420 = i8 3 items=["Stop"=-1, "Right translation"=6, "Back translation"=12, "Turning right"=0, "Turning left"=15, "Forward translation"=3, "Left translation"=9, "Gyro rotating"=16] ("Gait")
        # "物品架前对正"
        n183 = Index Array(array=w421) -> (element=w409:dbl)  [unwired: 1 in]
        n184 = Subtract(x=w409, y=93000.0) -> (x-y=w408:dbl)
        n185 = Increment(x=w423) -> (x+1=w422:u16)
        n186 = call "步态方向转换 (子VI).vi"("速度"=w408, "Gait"=w420) -> ("输出"=w419:dbl[])  [unwired: 9 in]
        n187 = call "PD.vi"("ENC"=w417, "SET"=w419) -> ("output"=w411:dbl[])  [unwired: 9 in]
        n188 = Less?(x=w411, y=0.5) -> (x < y?=w415:bool[])
        n189 = And Array Elements(Boolean array=w415) -> (logical AND=w414:bool)
        n190 = call "稳定T？.vi"("次数(100)"=30.0, "Reset"=w410, "输入"=w414) -> ("TT？"=w412:bool)  [unwired: 8 in]
        n191 = Select(t=w422, s=w412, f=w423) -> (s? t:f=w425:u16)
      }
      frame 29 {
        w432 = i8 6 items=["Stop"=-1, "Right translation"=6, "Back translation"=12, "Turning right"=0, "Turning left"=15, "Forward translation"=3, "Left translation"=9, "Gyro rotating"=16] ("Gait")
        # "货物架右扫线"
        n192 = call "步态方向转换 (子VI).vi"("速度"=15, "Gait"=w432) -> ("输出"=w430:dbl[])  [unwired: 9 in]
        n193 = Increment(x=w429) -> (x+1=w428:u16)
        n194 = Select(t=w428, s=w426, f=w429) -> (s? t:f=w427:u16)
      }
      frame 30 {
        # "松夹手"
        n195 = Index Array(array=w434, index=4 ("索引")) -> (element=w437:i32)
        n196 = Greater Or Equal?(x=w437, y=1300) -> (x >= y?=w435:bool)
        n197 = Increment(x=w440) -> (x+1=w433:u16)
        n198 = Select(t=w433, s=w435, f=w440) -> (s? t:f=w441:u16)
      }
      frame 31 {
        # "下抓手"
        n199 = Index Array(array=w445, index=5 ("索引")) -> (element=w448:i32)
        n200 = Greater Or Equal?(x=w448, y=14600) -> (x >= y?=w446:bool)
        n201 = Increment(x=w451) -> (x+1=w444:u16)
        n202 = Select(t=w444, s=w446, f=w451) -> (s? t:f=w452:u16)
      }
      frame 32 {
        # "夹托盘"
        n203 = Index Array(array=w456, index=4 ("索引")) -> (element=w459:i32)
        n204 = Less Or Equal?(x=w459, y=700) -> (x <= y?=w457:bool)
        n205 = Increment(x=w462) -> (x+1=w455:u16)
        n206 = Select(t=w455, s=w457, f=w462) -> (s? t:f=w463:u16)
      }
      frame 33 {
        # "起托盘"
        n207 = Index Array(array=w466, index=5 ("索引")) -> (element=w469:i32)
        n208 = Less Or Equal?(x=w469, y=10000) -> (x <= y?=w467:bool)
        n209 = Increment(x=w472) -> (x+1=w465:u16)
        n210 = Select(t=w465, s=w467, f=w472) -> (s? t:f=w473:u16)
      }
      frame 34 {
        w481 = i8 0 items=["Stop"=-1, "Right translation"=6, "Back translation"=12, "Turning right"=0, "Turning left"=15, "Forward translation"=3, "Left translation"=9, "Gyro rotating"=16] ("Gait")
        # "右转90"
        n211 = Greater?(x=w477, y=3500 ("次数")) -> (0:w483:bool[])
        n212 = Or Array Elements(Boolean array=w483) -> (logical OR=w482:bool)
        n213 = call "步态方向转换 (子VI).vi"("速度"=30, "Gait"=w481) -> ("输出"=w480:dbl[])  [unwired: 9 in]
        n214 = Increment(x=w479) -> (x+1=w478:u16)
        n215 = Select(t=w478, s=w482, f=w479) -> (s? t:f=w485:u16)
      }
      frame 35 {
        w494 = i8 3 items=["Stop"=-1, "Right translation"=6, "Back translation"=12, "Turning right"=0, "Turning left"=15, "Forward translation"=3, "Left translation"=9, "Gyro rotating"=16] ("Gait")
        # "前进到交付区"
        n216 = Greater?(x=w493, y=13000) -> (0:w490:bool[])
        n217 = Or Array Elements(Boolean array=w490) -> (logical OR=w487:bool)
        n218 = Increment(x=w488) -> (x+1=w489:u16)
        n219 = call "步态方向转换 (子VI).vi"("速度"=30, "Gait"=w494) -> ("输出"=w495:dbl[])  [unwired: 9 in]
        n220 = Select(t=w489, s=w487, f=w488) -> (s? t:f=w491:u16)
      }
      frame 36 {
        # "对正"
        n221 = feedback-in #5(w508) -> ()
        n222 = feedback #5() -> (w507:i32[])  [unwired: 1 in]
        n223 = Subtract(x=w508, y=w507) -> (x-y=w506:i32[])
        n224 = call "超声波对正(子VI).vi"("LFT"=120000.0, "FWD"=100000.0, "数组输入"=w513) -> ("数组输出"=w512:dbl[])  [unwired: 8 in]
        n225 = Increment(x=w511) -> (x+1=w496:u16)
        n226 = disable-structure shown="禁用" {
          disable-tunnel: w512 -> [w516 w517]
          disable-tunnel: [w514 w517] -> w509
          frame Disabled {
            n227 = call "限速.vi"("最大值"=60.0, "输入"=w516) -> ("数组"=w514:dbl[])  [unwired: 9 in]
          }
          frame Enabled {
          }
        }
        n228 = call "PD.vi"("ENC"=w506, "SET"=w509) -> ("output"=w505:dbl[])  [unwired: 9 in]
        n229 = Less?(x=w505, y=0.5) -> (x < y?=w503:bool[])
        n230 = And Array Elements(Boolean array=w503) -> (logical AND=w502:bool)
        n231 = call "稳定T？.vi"("次数(100)"=100.0, "Reset"=w500, "输入"=w502) -> ("TT？"=w501:bool)  [unwired: 8 in]
        n232 = Select(t=w496, s=w501, f=w511) -> (s? t:f=w510:u16)
      }
      frame 37 {
        # "下抓手"
        n233 = Index Array(array=w520, index=5 ("索引")) -> (element=w523:i32)
        n234 = Greater Or Equal?(x=w523, y=13000) -> (x >= y?=w521:bool)
        n235 = Increment(x=w526) -> (x+1=w519:u16)
        n236 = Select(t=w519, s=w521, f=w526) -> (s? t:f=w527:u16)
      }
      frame 38 {
        # "松夹手"
        n237 = Index Array(array=w530, index=4 ("索引")) -> (element=w533:i32)
        n238 = Greater Or Equal?(x=w533, y=1300) -> (x >= y?=w531:bool)
        n239 = Increment(x=w536) -> (x+1=w529:u16)
        n240 = Select(t=w529, s=w531, f=w536) -> (s? t:f=w537:u16)
      }
      frame 50 {
        n241 = Index Array(array=w539, index=4 ("索引")) -> (element=w542:i32)
        n242 = Less Or Equal?(x=w542, y=50) -> (x <= y?=w540:bool)
        n243 = Increment(x=w545) -> (x+1=w546:u16)
        n244 = Select(t=w546, s=w540, f=w545) -> (s? t:f=w547:u16)
      }
      frame 51 {
        n245 = Index Array(array=w551, index=5 ("索引")) -> (element=w554:i32)
        n246 = Less Or Equal?(x=w554, y=100) -> (x <= y?=w552:bool)
        n247 = Increment(x=w557) -> ()  [unwired: 1 out]
        n248 = Select(t=u16 0, s=w552, f=w557) -> (s? t:f=w558:u16)
      }
      frame 52 {
        w565 = i8 12 items=["Stop"=-1, "Right translation"=6, "Back translation"=12, "Turning right"=0, "Turning left"=15, "Forward translation"=3, "Left translation"=9, "Gyro rotating"=16] ("Gait")
        n249 = Greater?(x=w562, y=8000 ("长度 2")) -> (0:w563:bool[])
        n250 = Or Array Elements(Boolean array=w563) -> (logical OR=w561:bool)
        n251 = call "步态方向转换 (子VI).vi"("速度"=w560, "Gait"=w565) -> ("输出"=w566:dbl[])  [unwired: 9 in]
        n252 = Select(t=u16 0, s=w561, f=w568) -> (s? t:f=w569:u16)
      }
      frame 96 {
        # "抓"
        n253 = local read "货物类型"() -> (w572:dbl)
        n254 = Index Array(array=w573, index=4 ("索引")) -> (element=w576:i32)
        n255 = Quotient & Remainder(x=w572, y=2.0) -> (floor(x/y)=w570:dbl)  [unwired: 1 out]
        n256 = Equal To 0?(x=w570) -> ()  [unwired: 1 out]
        n257 = Less Or Equal?(x=w576, y=700) -> (x <= y?=w574:bool)
        n258 = Increment(x=w579) -> (x+1=w580:u16)
        n259 = Select(t=w580, s=w574, f=w579) -> (s? t:f=w581:u16)
      }
      frame 99 {
        # "货物类型判断"
        n260 = local read "大小"() -> (w586:dbl[])
        n261 = Array Max & Min(array=w586) -> (max value=w596:dbl, max index (indices)=w591:i32)  [unwired: 2 out]
        n262 = Greater Or Equal?(x=w596, y=50000.0 ("大小阈值")) -> (x >= y?=w597:bool)
        n263 = Select(t=1.0, s=w597, f=3.0) -> (s? t:f=w592:dbl)
        n264 = feedback #6() -> (w585:dbl)  [unwired: 1 in]
        n265 = Add(x=w592, y=w591) -> (x+y=w584:dbl)
        "货物类型" <- w584
        n266 = feedback-in #6(w584) -> ()
        n267 = Not Equal?(x=w584, y=w585) -> (x != y?=w583:bool)
        n268 = Increment(x=w587) -> (x+1=w588:u16)
        n269 = Select(t=w588, s=w583, f=w587) -> (s? t:f=w589:u16)
      }
      frame 100 {
        # "停止"
        n270 = local write "货物类型"(0.0 ("货物类型")) -> ()
      }
    }
    n271 = Select(t=FALSE, s=w32, f=w35) -> (s? t:f=w34:bool)
    n272 = call "缓起(子VI).vi"("缓起清零"=w34, "输入"=w56) -> ("输出"=w58:i32[])  [unwired: 9 in]
    n273 = Not(x=w54) -> (.not. x?=w53:bool)
    n274 = Select(t=u16 50, s="Reset", f=w39) -> (s? t:f=w38:u16)
    n275 = call "PID.vi"("继电器"=w53, "SET"=w58, "ENC"=w47) -> ("DIR"=w62:bool[], "PWM"=w63:dbl[])  [unwired: 7 in]
    n276 = call "DIR RT.vi"("DIR"=w62, "Custom FPGA Reference Out"=w45) -> ()  [unwired: 8 in, 2 out]
    n277 = call "PWM RT总.vi"("PWM"=w63, "Custom FPGA Reference Out"=w45) -> ()  [unwired: 8 in, 2 out]
    n278 = Select(t=u16 100 ("f"), s="停止", f=w38) -> (s? t:f=w42:u16)
    n279 = node-c288() -> ()  [unwired: 1 in, 1 out]
    n280 = local write "停止 2"(w43) -> ()
    "当前步态" <- w31
  }
  n281 = while {
    tunnel: w17 -> [w619]
    tunnel: w7 -> [w612]
    tunnel: w6 -> [w611]
    tunnel: w19 -> [w621]
    tunnel: [w620] -> w18
    tunnel: w5 -> [w607]
    tunnel: [w606] -> w4
    stop <- "停止 2" stop-if-true
    # "图像处理"
    n282 = Build Array(w612, w611) -> (w618:T2[])
    n283 = call <vilib>:"IMAQdx Grab2.vi"("Image In"=w619, "Session In"=w621) -> ("Image Out"=w613:T2, "Session Out"=w620:T1)  [unwired: 6 in, 2 out]
    n284 = for {
      tunnel: cluster{"Lower value":i32, "Upper value":i32}[] [{"Lower value"=220, "Upper value"=255}, {"Lower value"=0, "Upper value"=100}] -> [w647] mode=indexing
      tunnel: cluster{"Lower value":i32, "Upper value":i32}[] [{"Lower value"=0, "Upper value"=106}, {"Lower value"=75, "Upper value"=200}] -> [w646] mode=indexing
      tunnel: cluster{"Lower value":i32, "Upper value":i32}[] [{"Lower value"=5, "Upper value"=97}, {"Lower value"=170, "Upper value"=255}] -> [w645] mode=indexing
      tunnel: [w627] -> w614 mode=indexing
      tunnel: [w626] -> w610 mode=indexing
      tunnel: w613 -> [w625]
      tunnel: w618 -> [w624] mode=indexing
      tunnel: w607 -> [w623]
      tunnel: [w622] -> w606
      w633 = i32[] [] items=["Center of Mass X", "Center of Mass Y", "First Pixel X", "First Pixel Y", "Bounding Rect Left", "Bounding Rect Top", "Bounding Rect Right", "Bounding Rect Bottom", "Max Feret Diameter Start X", "Max Feret Diameter Start Y", "Max Feret Diameter End X", "Max Feret Diameter End Y", "Max Horiz. Segment Length Left", "Max Horiz. Segment Length Right", "Max Horiz. Segment Length Row", "-", "Bounding Rect Width", "Bounding Rect Height", "Bounding Rect Diagonal", "Perimeter", "Convex Hull Perimeter", "Holes' Perimeter", "Max Feret Diameter", "Equivalent Ellipse Major Axis", "Equivalent Ellipse Minor Axis", "Equivalent Ellipse Minor Axis (Feret)", "Equivalent Rect Long Side", "Equivalent Rect Short Side", "Equivalent Rect Diagonal", "Equivalent Rect Short Side (Feret)", "Average Horiz. Segment Length", "Average Vert. Segment Length", "Hydraulic Radius", "Waddel Disk Diameter", "-", "Area", "Holes' Area", "Particle & Holes' Area", "Convex Hull Area", "Image Area", "-", "Number of Holes", "Number of Horiz. Segments", "Number of Vert. Segments", "-", "Orientation", "Max Feret Diameter Orientation", "-", "% Area/Image Area", "% Area/(Particle & Holes' Area)", "Ratio of Equivalent Ellipse Axes", "Ratio of Equivalent Rect Sides", "-", "Elongation Factor", "Compactness Factor", "Heywood Circularity Factor", "Type Factor", "-", "Sum X", "Sum Y", "Sum XX", "Sum XY", "Sum YY", "Sum XXX", "Sum XXY", "Sum XYY", "Sum YYY", "-", "Moment of Inertia XX", "Moment of Inertia XY", "Moment of Inertia YY", "Moment of Inertia XXX", "Moment of Inertia XXY", "Moment of Inertia XYY", "Moment of Inertia YYY", "Norm. Moment of Inertia XX", "Norm. Moment of Inertia XY", "Norm. Moment of Inertia YY", "Norm. Moment of Inertia XXX", "Norm. Moment of Inertia XXY", "Norm. Moment of Inertia XYY", "Norm. Moment of Inertia YYY", "Hu Moment 1", "Hu Moment 2", "Hu Moment 3", "Hu Moment 4", "Hu Moment 5", "Hu Moment 6", "Hu Moment 7"] ("Real-World Measurements")
      w634 = i32[] [35] items=["Center of Mass X", "Center of Mass Y", "First Pixel X", "First Pixel Y", "Bounding Rect Left", "Bounding Rect Top", "Bounding Rect Right", "Bounding Rect Bottom", "Max Feret Diameter Start X", "Max Feret Diameter Start Y", "Max Feret Diameter End X", "Max Feret Diameter End Y", "Max Horiz. Segment Length Left", "Max Horiz. Segment Length Right", "Max Horiz. Segment Length Row", "-", "Bounding Rect Width", "Bounding Rect Height", "Bounding Rect Diagonal", "Perimeter", "Convex Hull Perimeter", "Holes' Perimeter", "Max Feret Diameter", "Equivalent Ellipse Major Axis", "Equivalent Ellipse Minor Axis", "Equivalent Ellipse Minor Axis (Feret)", "Equivalent Rect Long Side", "Equivalent Rect Short Side", "Equivalent Rect Diagonal", "Equivalent Rect Short Side (Feret)", "Average Horiz. Segment Length", "Average Vert. Segment Length", "Hydraulic Radius", "Waddel Disk Diameter", "-", "Area", "Holes' Area", "Particle & Holes' Area", "Convex Hull Area", "Image Area", "-", "Number of Holes", "Number of Horiz. Segments", "Number of Vert. Segments", "-", "Orientation", "Max Feret Diameter Orientation", "-", "% Area/Image Area", "% Area/(Particle & Holes' Area)", "Ratio of Equivalent Ellipse Axes", "Ratio of Equivalent Rect Sides", "-", "Elongation Factor", "Compactness Factor", "Heywood Circularity Factor", "Type Factor", "-", "Sum X", "Sum Y", "Sum XX", "Sum XY", "Sum YY", "Sum XXX", "Sum XXY", "Sum XYY", "Sum YYY", "-", "Moment of Inertia XX", "Moment of Inertia XY", "Moment of Inertia YY", "Moment of Inertia XXX", "Moment of Inertia XXY", "Moment of Inertia XYY", "Moment of Inertia YYY", "Norm. Moment of Inertia XX", "Norm. Moment of Inertia XY", "Norm. Moment of Inertia YY", "Norm. Moment of Inertia XXX", "Norm. Moment of Inertia XXY", "Norm. Moment of Inertia XYY", "Norm. Moment of Inertia YYY", "Hu Moment 1", "Hu Moment 2", "Hu Moment 3", "Hu Moment 4", "Hu Moment 5", "Hu Moment 6", "Hu Moment 7"] ("Pixel Measurements")
      w631 = TRUE ("Connectivity 4/8 (8)")
      w648 = u16 0 items=["RGB", "HSL", "HSV", "HSI"] ("Color Mode")
      n285 = call "IMAQ ColorThreshold"("Blue or Luma or Val or Inten Range"=w645, "Replace Value"=1, "Green or Sat Range"=w646, "Color Mode"=w648, "error in (no error)"=w623, "Red or Hue Range"=w647, "Image Dst"=w624, "Image Src"=w625) -> ("error out"=w644:errorcluster, "Image Dst Out"=w639:T2)  [unwired: 2 out]
      n286 = call "IMAQ RemoveParticle"("Connectivity 4/8 (8)"=TRUE, "Low Pass/High Pass (Low)"=FALSE, "Square/Hexa (Square)"=FALSE, "error in (no error)"=w644, "Number of Erosion"=5, "Image Src"=w639) -> ("error out"=w638:errorcluster, "Image Dst Out"=w636:T2)  [unwired: 1 in, 3 out]
      n287 = call "IMAQ FillHole"("error in (no error)"=w638, "Image Src"=w636, "Connectivity 4/8 (8)"=TRUE) -> ("error out"=w635:errorcluster, "Image Dst Out"=w632:T2)  [unwired: 1 in, 2 out]
      n288 = call "IMAQ Particle Analysis"("Connectivity 4/8 (8)"=w631, "error in (no error)"=w635, "Real-World Measurements"=w633, "Pixel Measurements"=w634, "Image"=w632) -> ("error out"=w628:errorcluster, "Particle Measurements (Pixels)"=w626:dbl[][], "Image Out (duplicate)"=w630:T2)  [unwired: 4 out]
      n289 = call <vilib>:"IVA Store Particles Results.vi"("error in (no error)"=w628, "Connectivity 4/8 (8)"=w631, "Step Name"="Particle Analysis 1", "Image in"=w630) -> ("error out"=w622:errorcluster, "Number of Particles"=w627:i32)  [unwired: 6 out]
    }
    "数量" <- w614
    n290 = Reshape Array(w610, 2 ("维数大小")) -> (→"大小":dbl[])
    n291 = Wait (ms)(milliseconds to wait=u32 5 ("等待时间（毫秒）")) -> ()  [unwired: 1 out]
  }
  n292 = call <vilib>:"IMAQdx Close Camera.vi"("error in"=w4, "Session In"=w18) -> ("error out"=w16:errorcluster)  [unwired: 9 in]
  n293 = Not(x="保留图像？") -> (.not. x?=w2:bool)
  n294 = call "IMAQ Dispose"("All Images? (No)"=w2, "error in (no error)"=w16) -> ()  [unwired: 4 in, 1 out]
  n295 = node-c288(w29) -> (w26:errorcluster)
  n296 = xnode "关闭FPGA VI引用"("FPGA VI引用输入"=w20, "错误输入"=w26) -> ("错误输出"=w25:errorcluster)
  n297 = call <vilib>:"Reset myRIO.vi"("error in (no error)"=w25) -> ()  [unwired: 10 in, 1 out]
